vi "NGTS_Filter Error Codes.vi"(8 "error in (no error)":errorcluster, 11 "Filter Error Codes":i32[](array[numeric])) -> (0 "error out":errorcluster)   [LabVIEW 2018]
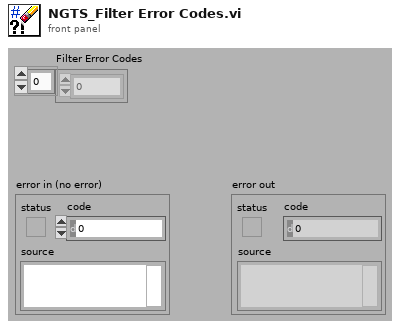
[diagram p1: front panel]
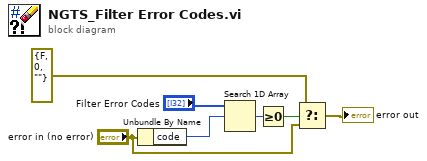
[diagram p0: block diagram]
diagram:
  n1 = Unbundle By Name("error in (no error)") -> ("code"=w6:i32)
  n2 = Search 1D Array(1D array="Filter Error Codes", element=w6) -> (index of element=w5:i32)  [unwired: 1 in]
  n3 = Greater Or Equal To 0?(x=w5) -> (x >= 0?=w4:bool)
  n4 = Select(t=errorcluster {"status"=FALSE, "code"=0, "source"=""}, s=w4, f="error in (no error)") -> (s? t:f=→"error out":errorcluster)
